vi "New Observing Viewable.vi"() -> (1 "Test Reply Queue":refnum<queue>, 3 "ObservingViewable out":refnum<class "ObservingViewable.lvclass">)   [LabVIEW 2015, in "ObservingViewable.lvclass"]
uses:
  ObservingViewable.lvclass
  ObservingViewable.lvclass/ObservingViewable.ctl
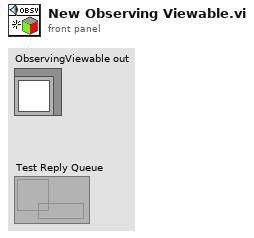
[diagram p1: front panel]
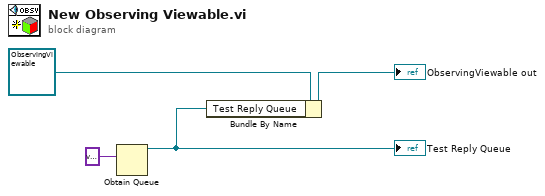
[diagram p0: block diagram]
diagram:
  n1 = Obtain Queue(element data type=variant) -> (queue out=w1:refnum<queue>)  [unwired: 4 in, 2 out]
  "Test Reply Queue" <- w1
  n2 = Bundle By Name(cluster=refnum<class "ObservingViewable.lvclass"> refnum ("ObservingViewable in"), "Test Reply Queue"=w1) -> (→"ObservingViewable out":refnum<class "ObservingViewable.lvclass">)
